vi "Argument Editor.vi"() -> ()   [LabVIEW 2020]
uses:
  LabVIEW 2020 Toolkits/toolkits_lv2020_32bit/Synchronization.llb/SynchRefs_SetGet.ctl
  LabVIEW 2020 Toolkits/VI Server Toolkit/VI Server Libraries/VI Server_GetControl.llb/VI Server_1D_Array_STR_Get.vi
  LabVIEW 2020 Toolkits/VI Server Toolkit/VI Server Libraries/VI Server_SetControl.llb/VI Server_1D_STR_Set.vi
  LabVIEW 2020 Toolkits/VI Server Toolkit/VI Server Libraries/VI Server_SetControl.llb/VI Server_I32_Set.vi
panel:
  in  "Export":bool
  in  "Removed.Indicator.Labels.Apply":bool
  in  "GET":string
  in  "RemovedLabels.[GET]":string[](array[string]) caption="Removed Indicator's Labels"
  in  "TargetVI.Indicators.Format[GET]":bool
  out "TargetVI.NumberOfIndicators":i32 caption="Number Of Indicators"
  in  "TargetVI.Indicators":string[](array[string]) caption="TargetVI Indicators"
  in  "TargetVI.Indicators.RemoveFromList":bool caption="Remove From List"
  in  "Removed.Control.Labels.Apply":bool
  in  "RemovedLabels":string[](array[string]) caption="Removed Labels"
  in  "Argument 3: Data Type":string caption="[Argument 3: Data Type]"
  in  "SET":string
  in  "TargetVI.Controls.Format[SET]":bool
  in  "TargetVI.Controls.RemoveFromList":bool caption="Remove From List"
  out "TargetVI.NumberOfControls":i32 caption="Number Of Controls"
  in  "TargetVI.Controls":string[](array[string]) caption="TargetVI Controls"
  in  "TabControls":string[](array[string]) caption="Tab Controls"
  in  "SourceVI.LOAD":bool
  in  "SourceVI":path caption="Source VI"
  in  "EXIT":bool
  out "error out":errorcluster
  in  "error in":errorcluster
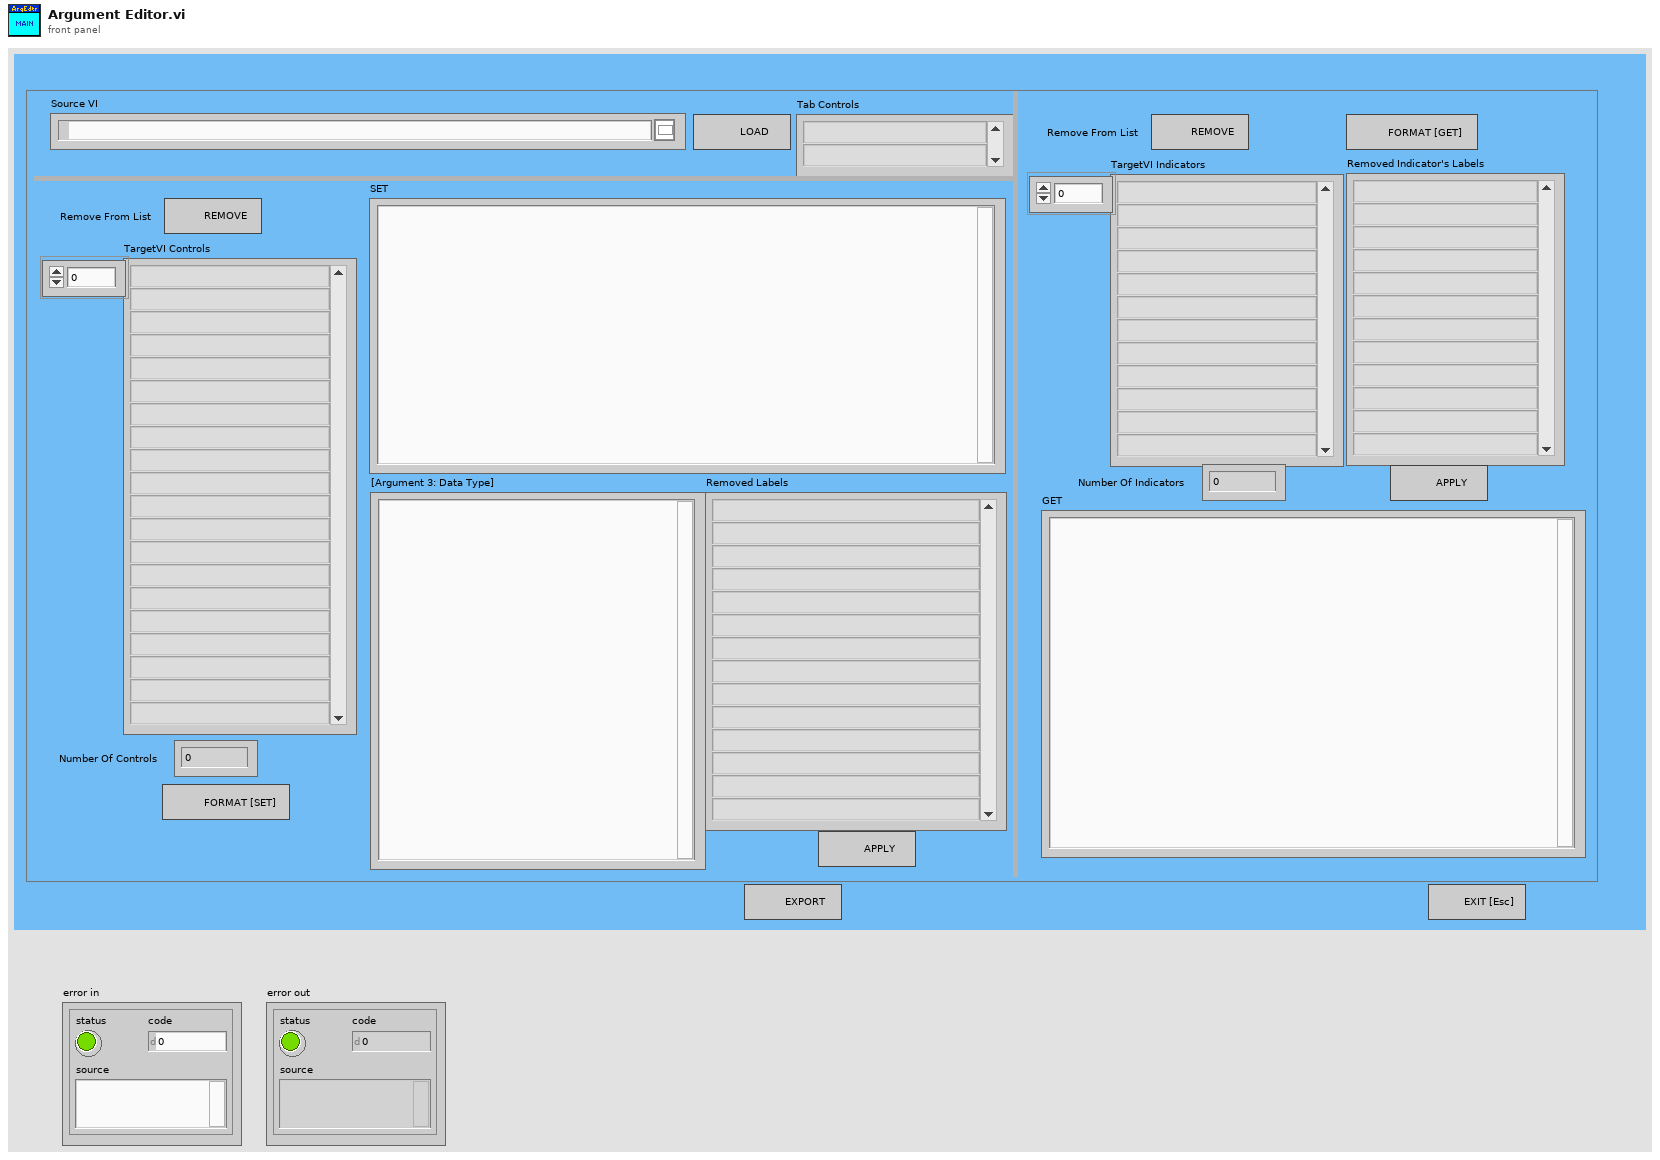
[diagram p1: front panel]
types:
  T1 = typedef "VI Server_RefsCluster.ctl" = cluster{"Labels":string[], "Refs":refnum<vi>[], "VI Ref":refnum<vi>}
  T2 = typedef "SynchRefs_SetGet.ctl" = enum16{"Set", "Get"}
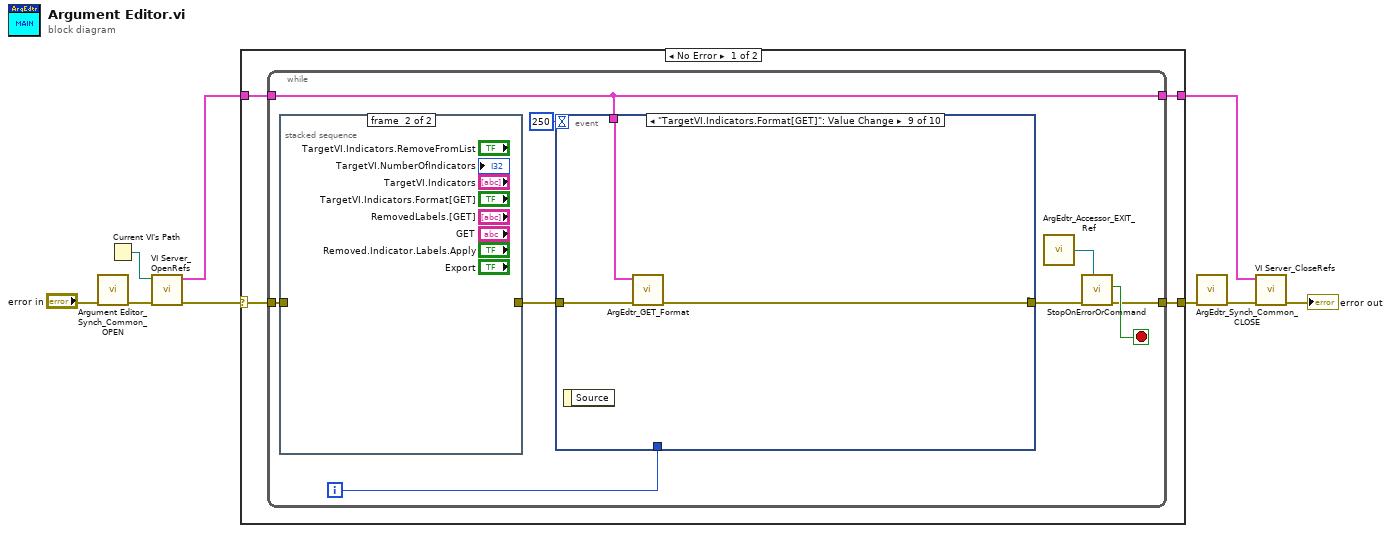
[diagram p0: block diagram]
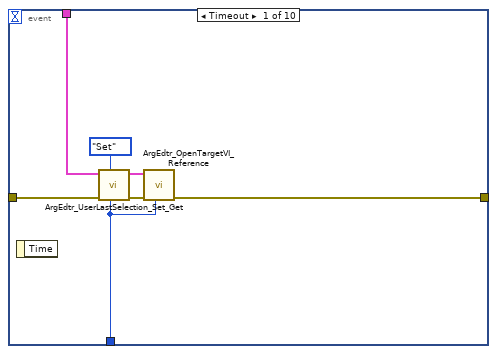
[diagram p2: hidden frame]
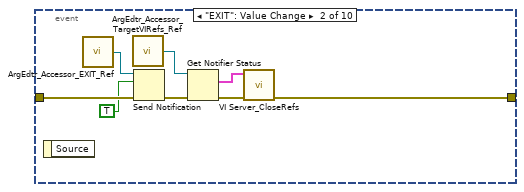
[diagram p3: hidden frame]
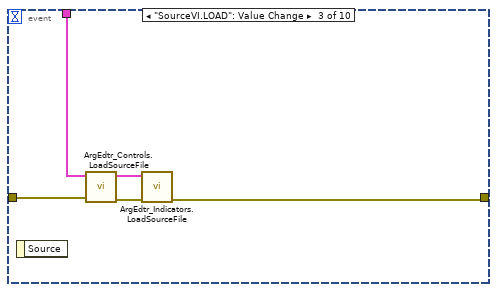
[diagram p4: hidden frame]
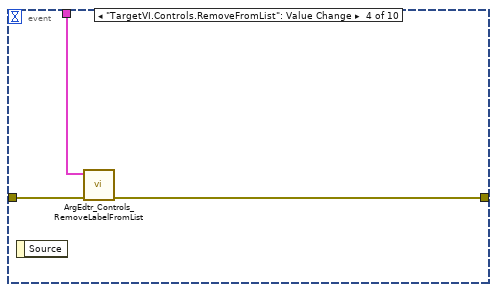
[diagram p5: hidden frame]
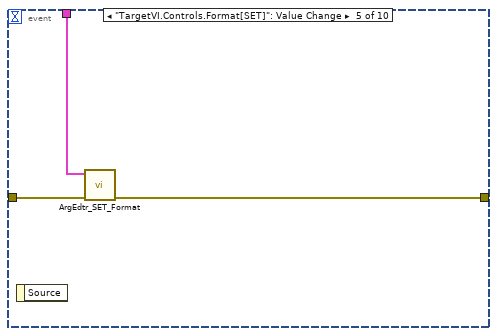
[diagram p6: hidden frame]
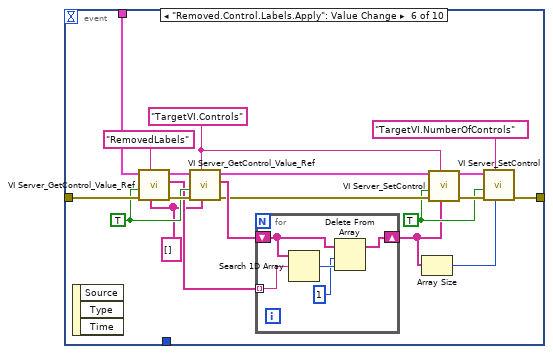
[diagram p7: hidden frame]
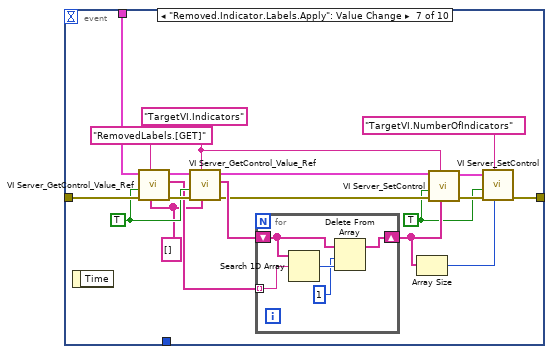
[diagram p8: hidden frame]
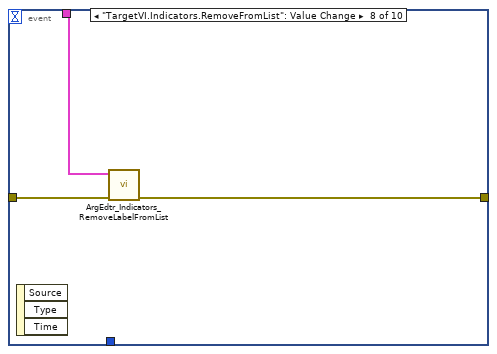
[diagram p9: hidden frame]
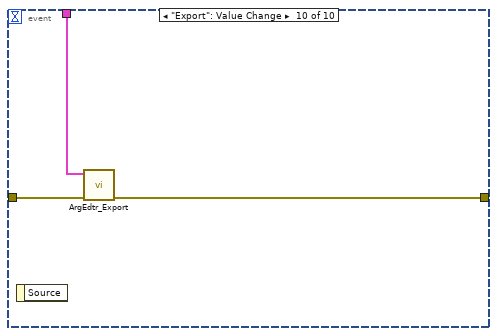
[diagram p10: hidden frame]
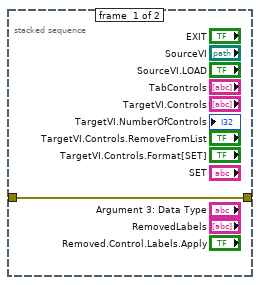
[diagram p11: hidden frame]
diagram:
  n1 = call "Argument Editor_Synch_Common_OPEN.vi"("error in (no error)"="error in") -> ("error out"=w7:errorcluster)  [unwired: 10 in]
  n2 = Current VI's Path() -> (path=w9:path)
  n3 = call "VI Server_OpenRefs.vi"("error in"=w7, "VI Path"=w9) -> ("error out"=w6:errorcluster, "VI Server.RefsCluster"=w5:T1)  [unwired: 8 in]
  n4 = case shown="No Error" w6 {
    selector: w6 -> [w12 w107]
    tunnel: w5 -> [w13 _]
    tunnel: [w11 w107] -> w4
    tunnel: [w10 _] -> w1
    frame No Error {
      n5 = while {
        tunnel: w13 -> [w15]
        tunnel: w12 -> [w22]
        tunnel: [w17] -> w11
        tunnel: [w15] -> w10
        i -> [w14]
        stop <- w18 stop-if-true
        n6 = stacked-sequence {
          tunnel: w22 -> [w106 _]
          tunnel: [w106 _] -> w21
          frame #0 {
          }
          frame #1 {
          }
        }
        n7 = event shown="[8] \"TargetVI.Indicators.Format[GET]\": Value Change" {
          selector: _ -> [_ _ _ _ _ _ _ _ _ _]
          dyn-events: _ -> [_ _ _ _ _ _ _ _ _ _]
          timeout: 250 -> [_ _ _ _ _ _ _ _ _ _]
          tunnel: w21 -> [w29 w37 w42 w45 w48 w67 w91 w99 w102 w105]
          tunnel: [w25 w31 w39 w43 w47 w53 w77 w97 w100 w104] -> w19
          tunnel: w15 -> [w28 _ w41 w44 w46 w66 w90 w98 w101 w103]
          tunnel: w14 -> [w23 _ _ _ _ _ _ _ _ _]
          event Timeout {
            n8 = event-data() -> ()  [unwired: 1 in, 1 out]
            n9 = call "ArgEdtr_UserLastSelection_Set_Get.vi"("LoopCounter"=w23, "SynchRefs.Set/Get"=SynchRefs_SetGet."Set", "error in"=w29, "VI Server.RefsCluster"=w28) -> ("error out"=w26:errorcluster, "VI Server.RefsCluster.DUP"=w24:T1)  [unwired: 6 in]
            n10 = call "ArgEdtr_OpenTargetVI_Reference.vi"("LoopCounter"=w23, "error in (no error)"=w26, "VI Server.RefsCluster"=w24) -> ("error out"=w25:errorcluster)  [unwired: 8 in]
          }
          event "EXIT": Value Change {
            n11 = event-data() -> ()  [unwired: 1 in, 1 out]
            n12 = call "ArgEdtr_Accessor_EXIT_Ref.vi"() -> ("EXIT"=w36:refnum<notifier>)  [unwired: 6 in]
            n13 = call "ArgEdtr_Accessor_TargetVIRefs_Ref.vi"() -> ("TargetVIServerRef"=w33:refnum<notifier>)  [unwired: 6 in]
            n14 = Send Notification(notification=TRUE, notifier=w36, error in (no error)=w37) -> (error out=w34:errorcluster)  [unwired: 1 out]
            n15 = Get Notifier Status(notifier=w33, error in (no error)=w34) -> (current notification=w30:T1, error out=w32:errorcluster)  [unwired: 3 out]
            n16 = call "VI Server_CloseRefs.vi"("error in"=w32, "VI Server.RefsCluster"=w30) -> ("error out"=w31:errorcluster)  [unwired: 9 in]
          }
          event "SourceVI.LOAD": Value Change {
            n17 = event-data() -> ()  [unwired: 1 in, 1 out]
            n18 = call "ArgEdtr_Controls.LoadSourceFile.vi"("error in (no error)"=w42, "VI Server.RefsCluster"=w41) -> ("error out"=w40:errorcluster, "VI Server.RefsCluster.DUP"=w38:T1)  [unwired: 8 in]
            n19 = call "ArgEdtr_Indicators.LoadSourceFile.vi"("error in (no error)"=w40, "VI Server.RefsCluster"=w38) -> ("error out"=w39:errorcluster)  [unwired: 9 in]
          }
          event "TargetVI.Controls.RemoveFromList": Value Change {
            n20 = event-data() -> ()  [unwired: 1 in, 1 out]
            n21 = call "ArgEdtr_Controls_RemoveLabelFromList.vi"("error in (no error)"=w45, "VI Server.RefsCluster"=w44) -> ("error out"=w43:errorcluster)  [unwired: 9 in]
          }
          event "TargetVI.Controls.Format[SET]": Value Change {
            n22 = event-data() -> ()  [unwired: 1 in, 1 out]
            n23 = call "ArgEdtr_SET_Format.vi"("error in (no error)"=w48, "VI Server.RefsCluster"=w46) -> ("error out"=w47:errorcluster)  [unwired: 9 in]
          }
          event "Removed.Control.Labels.Apply": Value Change {
            w52 = TRUE ("SingleInstance")
            w60 = string[] []
            w56 = "TargetVI.Controls" ("Control.Label")
            w62 = TRUE ("SingleInstance")
            n24 = event-data() -> ()  [unwired: 1 in, 3 out]
            n25 = call-poly "VI Server_GetControl_Value_Ref.vi"("DataType"=w60, "Control.Label"="RemovedLabels", "error in"=w67, "SingleInstance"=w62, "VI Server.RefsCluster"=w66) -> ("error out"=w64:errorcluster, "Value"=w61:string[], "VI Server.RefsCluster.DUP"=w63:T1)  [unwired: 3 in, 1 out]
            n26 = call-poly "VI Server_GetControl_Value_Ref.vi"("DataType"=w60, "Control.Label"=w56, "error in"=w64, "SingleInstance"=w62, "VI Server.RefsCluster"=w63) -> ("error out"=w57:errorcluster, "Value"=w59:string[], "VI Server.RefsCluster.DUP"=w58:T1)  [unwired: 3 in, 1 out]
            n27 = for {
              tunnel: w61 -> [w72] mode=indexing
              shift-right: [w68] -> w51
              shift-left: w59 -> [w69]
              n28 = Search 1D Array(1D array=w69, element=w72) -> (index of element=w71:i32)  [unwired: 1 in]
              n29 = Delete From Array(array=w69, length=1, index=w71) -> (array with subset deleted=w68:string[])  [unwired: 1 out]
            }
            n30 = Array Size(array=w51) -> (size(s)=w50:i32)
            n31 = call-poly "VI Server_SetControl.vi"("Data"=w51, "Control.Label"=w56, "error in"=w57, "SingleInstance"=w52, "VI Server.RefsCluster"=w58) -> ("error out"=w54:errorcluster, "VI Server.RefsCluster.DUP"=w55:T1)  [unwired: 4 in, 1 out]
            n32 = call-poly "VI Server_SetControl.vi"("Data"=w50, "Control.Label"="TargetVI.NumberOfControls", "error in"=w54, "SingleInstance"=w52, "VI Server.RefsCluster"=w55) -> ("error out"=w53:errorcluster)  [unwired: 4 in, 2 out]
          }
          event "Removed.Indicator.Labels.Apply": Value Change {
            w75 = TRUE ("SingleInstance")
            w84 = string[] []
            w80 = "TargetVI.Indicators" ("Control.Label")
            w86 = TRUE ("SingleInstance")
            n33 = event-data() -> ()  [unwired: 1 in, 1 out]
            n34 = call-poly "VI Server_GetControl_Value_Ref.vi"("DataType"=w84, "Control.Label"="RemovedLabels.[GET]", "error in"=w91, "SingleInstance"=w86, "VI Server.RefsCluster"=w90) -> ("error out"=w88:errorcluster, "Value"=w85:string[], "VI Server.RefsCluster.DUP"=w87:T1)  [unwired: 3 in, 1 out]
            n35 = call-poly "VI Server_GetControl_Value_Ref.vi"("DataType"=w84, "Control.Label"=w80, "error in"=w88, "SingleInstance"=w86, "VI Server.RefsCluster"=w87) -> ("error out"=w81:errorcluster, "Value"=w83:string[], "VI Server.RefsCluster.DUP"=w82:T1)  [unwired: 3 in, 1 out]
            n36 = for {
              tunnel: w85 -> [w96] mode=indexing
              shift-right: [w92] -> w79
              shift-left: w83 -> [w93]
              n37 = Search 1D Array(1D array=w93, element=w96) -> (index of element=w95:i32)  [unwired: 1 in]
              n38 = Delete From Array(array=w93, length=1, index=w95) -> (array with subset deleted=w92:string[])  [unwired: 1 out]
            }
            n39 = Array Size(array=w79) -> (size(s)=w74:i32)
            n40 = call-poly "VI Server_SetControl.vi"("Data"=w79, "Control.Label"=w80, "error in"=w81, "SingleInstance"=w75, "VI Server.RefsCluster"=w82) -> ("error out"=w78:errorcluster, "VI Server.RefsCluster.DUP"=w76:T1)  [unwired: 4 in, 1 out]
            n41 = call-poly "VI Server_SetControl.vi"("Data"=w74, "Control.Label"="TargetVI.NumberOfIndicators", "error in"=w78, "SingleInstance"=w75, "VI Server.RefsCluster"=w76) -> ("error out"=w77:errorcluster)  [unwired: 4 in, 2 out]
          }
          event "TargetVI.Indicators.RemoveFromList": Value Change {
            n42 = event-data() -> ()  [unwired: 1 in, 3 out]
            n43 = call "ArgEdtr_Indicators_RemoveLabelFromList.vi"("error in (no error)"=w99, "VI Server.RefsCluster"=w98) -> ("error out"=w97:errorcluster)  [unwired: 9 in]
          }
          event "TargetVI.Indicators.Format[GET]": Value Change {
            n44 = event-data() -> ()  [unwired: 1 in, 1 out]
            n45 = call "ArgEdtr_GET_Format.vi"("error in (no error)"=w102, "VI Server.RefsCluster"=w101) -> ("error out"=w100:errorcluster)  [unwired: 9 in]
          }
          event "Export": Value Change {
            n46 = event-data() -> ()  [unwired: 1 in, 1 out]
            n47 = call "ArgEdtr_Export.vi"("error in (no error)"=w105, "VI Server.RefsCluster"=w103) -> ("error out"=w104:errorcluster)  [unwired: 9 in]
          }
        }
        n48 = call "ArgEdtr_Accessor_EXIT_Ref.vi"() -> ("EXIT"=w16:refnum<notifier>)  [unwired: 6 in]
        n49 = call "StopOnErrorOrCommand.vi"("STOP"=w16, "error in (no error)"=w19) -> ("error out"=w17:errorcluster, "STOP"=w18:bool)  [unwired: 8 in]
      }
    }
    frame Error {
    }
  }
  n50 = call "ArgEdtr_Synch_Common_CLOSE.vi"("error in (no error)"=w4) -> ("error out"=w3:errorcluster)  [unwired: 10 in]
  n51 = call "VI Server_CloseRefs.vi"("error in"=w3, "VI Server.RefsCluster"=w1) -> ("error out"=→"error out":errorcluster)  [unwired: 9 in]
